vi "Teardown.vi"(8 "error in (no error)":errorcluster, 11 "Environment.LogFile in":refnum<class "Environment.LogFile.lvclass">) -> (0 "error out":errorcluster, 3 "Environment.LogFile out":refnum<class "Environment.LogFile.lvclass">)   [LabVIEW 2018, in "Environment.LogFile.lvclass"]
uses:
  Environment.LogFile.lvclass
  Environment.LogFile.lvclass/Environment.LogFile.ctl
panel:
  # "Connector Pane"
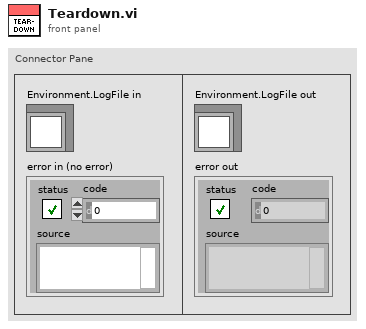
[diagram p1: front panel]
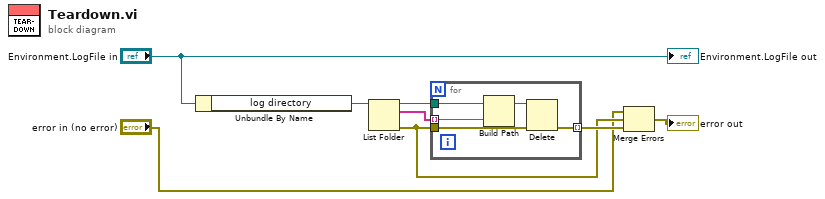
[diagram p0: block diagram]
diagram:
  n1 = Unbundle By Name("Environment.LogFile in") -> ("log directory"=w6:path)
  n2 = List Folder(path=w6) -> (path out=w5:path, filenames=w4:string[], error out=w3:errorcluster)  [unwired: 3 in, 1 out]
  n3 = for {
    tunnel: w5 -> [w9]
    tunnel: w3 -> [w13]
    tunnel: [w12] -> w8 mode=indexing
    tunnel: w4 -> [w10] mode=indexing
    n4 = Build Path(base path=w9, name or relative path=w10) -> (appended path=w11:path)
    n5 = Delete(path (use dialog)=w11, error in=w13) -> (error out=w12:errorcluster)  [unwired: 3 in, 2 out]
  }
  n6 = Merge Errors("error in (no error)", w3, w8) -> (→"error out":errorcluster)
  "Environment.LogFile out" <- "Environment.LogFile in"
